vi "MSEditor_ProcessFmtFGV.vi"(6 "Function":enum16{"Write", "Read"}(ring)=enum."Read", 7 "Script in":T1, 8 "error in (no error)":errorcluster, 9 "Ion trap":cluster{"R0":ext, "Z0":ext}, 10 "PriRF":T2, 11 "MS ProcessFMTs in":cluster{"ProcessName":string, "Data":variant}[](array[cluster])) -> (0 "error out":errorcluster, 1 "Ion trap out":cluster{"R0":ext, "Z0":ext}, 2 "PriRF out":T2, 3 "MS ProcessFMTs out":cluster{"ProcessName":string, "Data":variant}[](array[cluster]), 5 "Script out":T1)   [LabVIEW 2018]
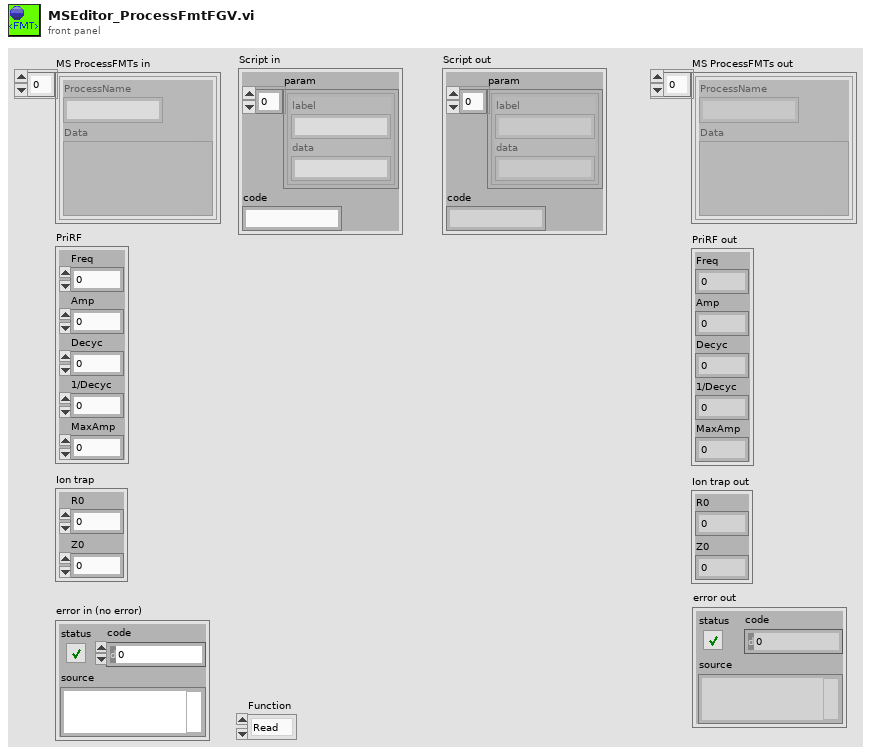
[diagram p1: front panel]
types:
  T1 = cluster{"param":cluster{"label":string, "data":string}[], "code":string}
  T2 = cluster{"Freq":ext, "Amp":ext, "Decyc":u32, "1/Decyc":u32, "MaxAmp":ext}
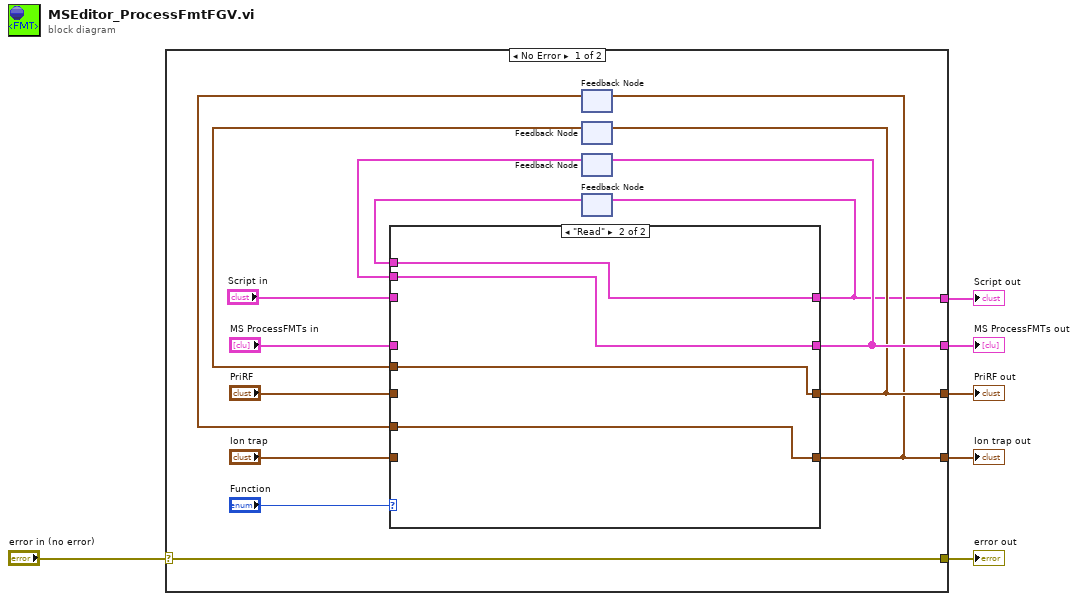
[diagram p0: block diagram]
diagram:
  n1 = case shown="No Error" "error in (no error)" {
    selector: "error in (no error)" -> [w10 w29]
    tunnel: [w19 _] -> w6
    tunnel: [w15 _] -> w5
    tunnel: [w13 _] -> w4
    tunnel: [w10 w29] -> w2
    tunnel: [w8 _] -> w1
    frame No Error {
      n2 = feedback #1() -> (w11:cluster{"R0":ext, "Z0":ext})  [unwired: 1 in]
      n3 = feedback #2() -> (w12:T2)  [unwired: 1 in]
      n4 = feedback #3() -> (w18:cluster{"ProcessName":string, "Data":variant}[])  [unwired: 1 in]
      n5 = feedback #4() -> (w9:T1)  [unwired: 1 in]
      n6 = case shown="\"Read\"" "Function" {
        tunnel: "MS ProcessFMTs in" -> [w24 _]
        tunnel: [w24 w28] -> w19
        tunnel: w18 -> [_ w28]
        tunnel: "PriRF" -> [w23 _]
        tunnel: [w23 w27] -> w15
        tunnel: "Ion trap" -> [w22 _]
        tunnel: [w22 w26] -> w13
        tunnel: w12 -> [_ w27]
        tunnel: w11 -> [_ w26]
        tunnel: "Script in" -> [w21 _]
        tunnel: [w21 w25] -> w8
        tunnel: w9 -> [_ w25]
        frame "Write", Default {
        }
        frame "Read" {
        }
      }
      n7 = feedback-in #1(w13) -> ()
      n8 = feedback-in #2(w15) -> ()
      n9 = feedback-in #3(w19) -> ()
      n10 = feedback-in #4(w8) -> ()
    }
    frame Error {
    }
  }
  "error out" <- w2
  "MS ProcessFMTs out" <- w6
  "Ion trap out" <- w4
  "PriRF out" <- w5
  "Script out" <- w1
